vi "Execute.vi"(11 "Sound Demo in":refnum<class "Sound Demo.lvclass">) -> (0 "error out":errorcluster, 3 "Sound Demo out":refnum<class "Sound Demo.lvclass">)   [LabVIEW 2010, in "Sound Demo.lvclass"]
doc: "Play a series of sounds on the chosen sound player."
uses:
  Sound Demo.lvclass
  Sound/Sound.lvclass
  Sound Demo.lvclass/Sound Demo.ctl
  Sound Player/Sound Player.lvclass
  <vilib>/Utility/xml.llb/Read From XML File(string).vi
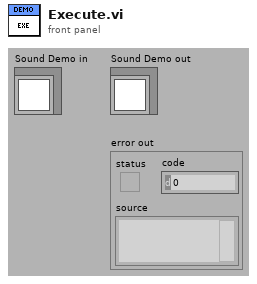
[diagram p1: front panel]
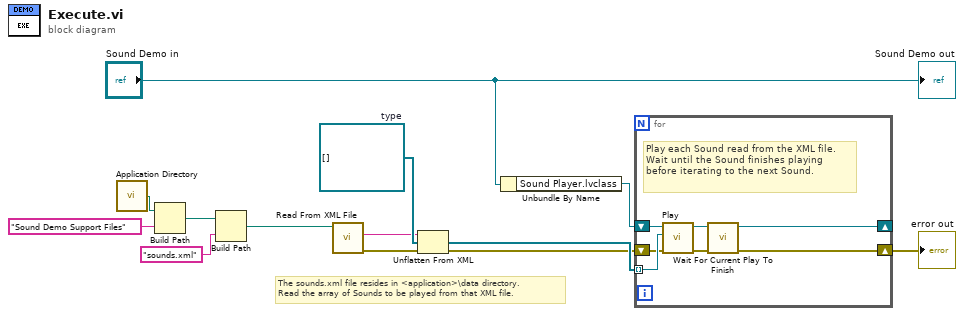
[diagram p0: block diagram]
diagram:
  w4 = refnum<class "Sound.lvclass">[] []  # type
  # "The sounds.xml file resides in <application>\\data directory.\nRead the array of Sounds to be played from that XML file."
  n1 = call <vilib>:"Application Directory.vi"() -> ("Application Directory"=w8:path)
  n2 = Build Path(base path=w8, name or relative path="Sound Demo Support Files") -> (appended path=w6:path)
  n3 = Build Path(base path=w6, name or relative path="sounds.xml") -> (appended path=w3:path)
  n4 = call-poly <vilib>:"Read From XML File.vi"("XML File Path"=w3) -> ("error out"=w1:errorcluster, "XML Elements"=w2:string)  [unwired: 8 in, 1 out]
  n5 = Unflatten From XML(xml string=w2, type=w4, error in (no error)=w1) -> (value=w10:refnum<class "Sound.lvclass">[], error out=w9:errorcluster)
  n6 = Unbundle By Name "Unbundle By Name"("Sound Demo in") -> ("Sound Player.lvclass"=w12:refnum<class "Sound Player.lvclass">)
  n7 = for {
    tunnel: w10 -> [w19] mode=indexing
    shift-right: [w16] -> _
    shift-left: w12 -> [w20]
    shift-right: [w14] -> w11
    shift-left: w9 -> [w18]
    # "Play each Sound read from the XML file. Wait until the Sound finishes playing before iterating to the next Sound."
    n8 = call-dynamic "Play.vi"("error in (no error)"=w18, "Sound"=w19, "Sound Player"=w20) -> ("error out"=w15:errorcluster, "Sound Player out"=w17:refnum<class "Sound Player.lvclass">)  [unwired: 7 in]
    n9 = call "Wait For Current Play To Finish.vi"("error in (no error)"=w15, "Sound Player in"=w17) -> ("error out"=w14:errorcluster, "Sound Player out"=w16:refnum<class "Sound Player.lvclass">)  [unwired: 8 in]
  }
  "error out" <- w11
  "Sound Demo out" <- "Sound Demo in"
